vi "FTW-Test-JSON-ElementInfo.vi"() -> (0 "Test Result":errorcluster)   [LabVIEW 2015]
uses:
  src/json/FTW-JSON-Type.ctl
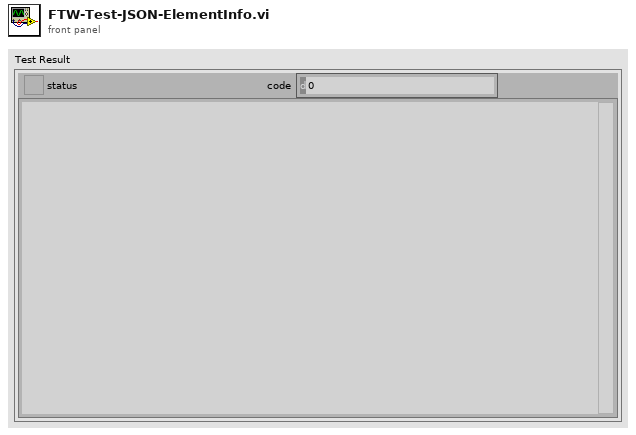
[diagram p1: front panel]
types:
  T1 = typedef "FTW-JSON-Type.ctl" = enum8{"Not Found", "Object", "Array", "String", "Number", "Boolean", "null"}
  T2 = cluster{"Path":string, "NumElements":i32, "ExpectedType":T1}[]
  T3 = typedef "FTW-Type-JSON.ctl" = refnum<data-value>
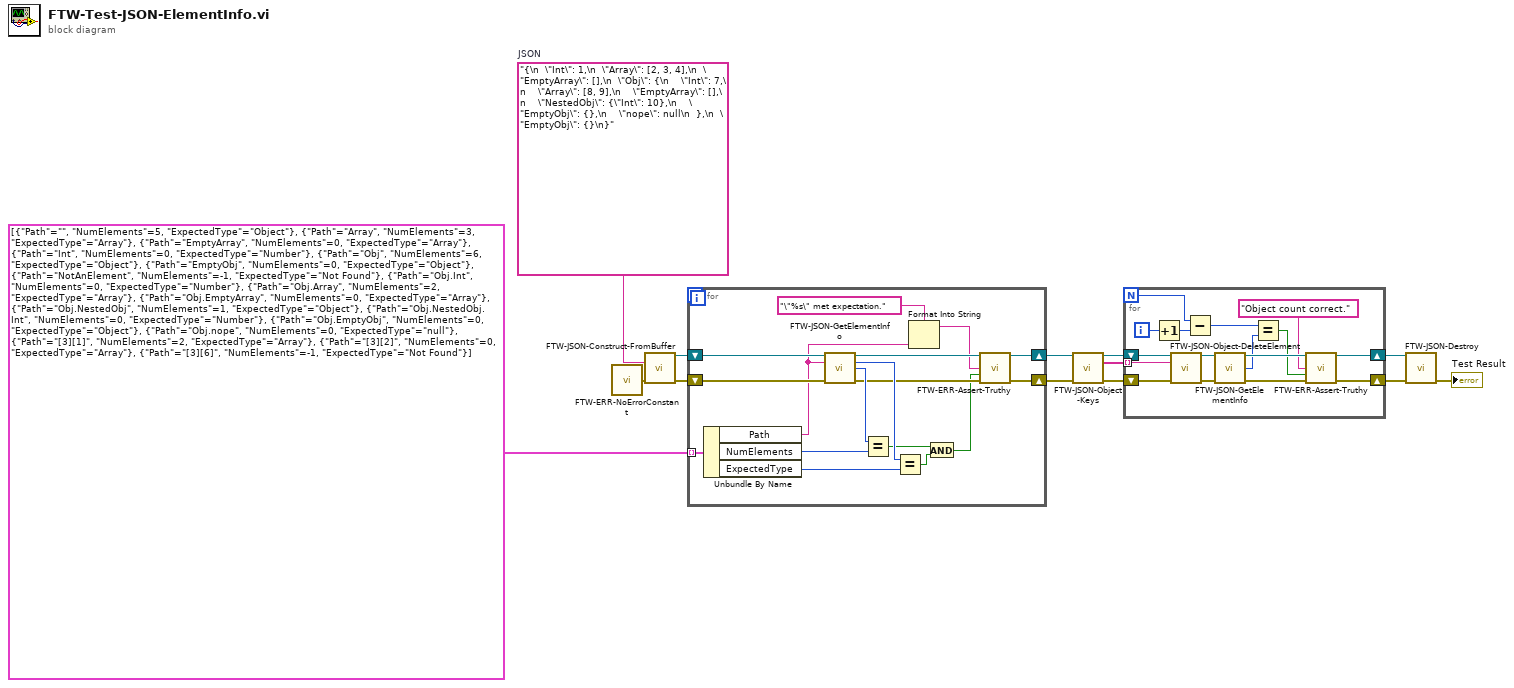
[diagram p0: block diagram]
diagram:
  w8 = "{\n  \"Int\": 1,\n  \"Array\": [2, 3, 4],\n  \"EmptyArray\": [],\n  \"Obj\": {\n    \"Int\": 7,\n    \"Array\": [8, 9],\n    \"EmptyArray\": [],\n    \"NestedObj\": {\"Int\": 10},\n    \"EmptyObj\": {},\n    \"nope\": null\n  },\n  \"EmptyObj\": {}\n}"  # JSON
  n1 = call "FTW-ERR-NoErrorConstant.vi"() -> ("no error"=w13:errorcluster)
  n2 = call "FTW-JSON-Construct-FromBuffer.vi"("JSON String (UTF-8)"=w8, "error in"=w13) -> ("JSON"=w7:T3, "error out"=w6:errorcluster)  [unwired: 12 in]
  n3 = for {
    shift-right: [w20] -> w3
    shift-left: w6 -> [w28]
    shift-right: [w27] -> w4
    shift-left: w7 -> [w29]
    tunnel: T2 [{"Path"="", "NumElements"=5, "ExpectedType"=enum."Object"}, {"Path"="Array", "NumElements"=3, "ExpectedType"=enum."Array"}, {"Path"="EmptyArray", "NumElements"=0, "ExpectedType"=enum."Array"}, {"Path"="Int", "NumElements"=0, "ExpectedType"=enum."Number"}, {"Path"="Obj", "NumElements"=6, "ExpectedType"=enum."Object"}, {"Path"="EmptyObj", "NumElements"=0, "ExpectedType"=enum."Object"}, {"Path"="NotAnElement", "NumElements"=-1, "ExpectedType"=enum."Not Found"}, {"Path"="Obj.Int", "NumElements"=0, "ExpectedType"=enum."Number"}, {"Path"="Obj.Array", "NumElements"=2, "ExpectedType"=enum."Array"}, {"Path"="Obj.EmptyArray", "NumElements"=0, "ExpectedType"=enum."Array"}, {"Path"="Obj.NestedObj", "NumElements"=1, "ExpectedType"=enum."Object"}, {"Path"="Obj.NestedObj.Int", "NumElements"=0, "ExpectedType"=enum."Number"}, {"Path"="Obj.EmptyObj", "NumElements"=0, "ExpectedType"=enum."Object"}, {"Path"="Obj.nope", "NumElements"=0, "ExpectedType"=enum."null"}, {"Path"="[3][1]", "NumElements"=2, "ExpectedType"=enum."Array"}, {"Path"="[3][2]", "NumElements"=0, "ExpectedType"=enum."Array"}, {"Path"="[3][6]", "NumElements"=-1, "ExpectedType"=enum."Not Found"}] -> [w25] mode=indexing
    n4 = Unbundle By Name(w25) -> ("Path"=w19:string, "NumElements"=w24:i32, "ExpectedType"=w22:T1)
    n5 = call "FTW-JSON-GetElementInfo.vi"("JSON"=w29, "Path to Element"=w19, "error in"=w28) -> ("JSON out"=w27:T3, "Element Type"=w23:T1, "Contained Elements"=w26:i32, "error out"=w21:errorcluster)  [unwired: 9 in]
    n6 = Equal?(x=w26, y=w24) -> (x = y?=w16:bool)
    n7 = Equal?(x=w23, y=w22) -> (x = y?=w15:bool)
    n8 = Format Into String(format string="\"%s\" met expectation.", w19) -> (resulting string=w17:string)  [unwired: 2 in, 1 out]
    n9 = And(x=w16, y=w15) -> (x .and. y?=w14:bool)
    n10 = call "FTW-ERR-Assert-Truthy.vi"("Assertion"=w17, "Assertion holds true?"=w14, "error in"=w21) -> ("error out"=w20:errorcluster)  [unwired: 12 in]
  }
  n11 = call "FTW-JSON-Object-Keys.vi"("JSON"=w4, "error in"=w3) -> ("JSON out"=w12:T3, "Keys"=w11:string[], "error out"=w10:errorcluster)  [unwired: 11 in]
  n12 = for {
    N -> [w37]
    tunnel: w11 -> [w42] mode=indexing
    shift-right: [w30] -> w1
    shift-left: w10 -> [w43]
    shift-right: [w40] -> w2
    shift-left: w12 -> [w44]
    i -> [w36]
    n13 = Increment(x=w36) -> (x+1=w35:i32)
    n14 = call "FTW-JSON-Object-DeleteElement.vi"("JSON"=w44, "Key"=w42, "error in"=w43) -> ("JSON out"=w41:T3, "error out"=w39:errorcluster)  [unwired: 10 in, 1 out]
    n15 = Subtract(x=w37, y=w35) -> (x-y=w34:i32)
    n16 = call "FTW-JSON-GetElementInfo.vi"("JSON"=w41, "error in"=w39) -> ("JSON out"=w40:T3, "Contained Elements"=w33:i32, "error out"=w31:errorcluster)  [unwired: 10 in, 1 out]
    n17 = Equal?(x=w34, y=w33) -> (x = y?=w32:bool)
    n18 = call "FTW-ERR-Assert-Truthy.vi"("Assertion"="Object count correct.", "Assertion holds true?"=w32, "error in"=w31) -> ("error out"=w30:errorcluster)  [unwired: 12 in]
  }
  n19 = call "FTW-JSON-Destroy.vi"("JSON"=w2, "error in"=w1) -> ("error out"=→"Test Result":errorcluster)  [unwired: 13 in]
